vi "SpecAn ACP Configure.vi"(7 "Selector String":string, 8 "error in (no error)":errorcluster, 10 "ACP Common Configuration":T1={"Power Units"=0, "Averaging Enabled"=0, "Averaging Count"=10, "Averaging Type"=0, "FFT Window"=1, "FFT Padding"=1.0, "RBW Auto"=1, "RBW (Hz)"=10000.0, "RBW Filter Type"=1, "Sweep Time Auto"=1, "Sweep Time Interval (s)"=0.001, " Carrier Channel Configuration"=[], "Offset Channel Configuration"=[]} {"Offset Channel Configuration"."RRC Alpha" format="%.3g"; "Offset Channel Configuration"."RRC Enabled" items=["False", "True"]; "Offset Channel Configuration"."Relative Attenuation (dB)" format="%.2f"; "Offset Channel Configuration"."Offset Power Reference Carrier" items=["Closest", "Highest", "Composite", "Specific"]; "Offset Channel Configuration"."Offset Sideband" items=["Neg", "Pos", "Both"]; "Offset Channel Configuration"."Offset Frequency (Hz)" format="%.3p"; "Offset Channel Configuration"."Offset Enabled" items=["False", "True"]; "Offset Channel Configuration"."Integration Bandwidth (Hz)" format="%.3p"; "Carrier Channel Configuration"."RRC Alpha" format="%.3g"; "Carrier Channel Configuration"."RRC Enabled" items=["False", "True"]; "Carrier Channel Configuration"."Mode" items=["Passive", "Active"]; "Carrier Channel Configuration"."Frequency (Hz)" format="%.3p"; "Carrier Channel Configuration"."Integration Bandwidth (Hz)" format="%.3p"; "Sweep Time Interval (s)" format="%.2p"; "Sweep Time Auto" items=["False", "True"]; "RBW Filter Type" items=["FFT Based", "Gaussian", "Flat", "Synch Tuned - 4", "Synch Tuned - 5"]; "RBW (Hz)" format="%.3p"; "RBW Auto" items=["False", "True"]; "FFT Padding" format="%.2p"; "FFT Window" items=["None", "Flat Top", "Hanning", "Hamming", "Gaussian", "Blackman", "Blackman-Harris", "Kaiser-Bessel"]; "Averaging Type" items=["RMS", "Log", "Scalar", "Max", "Min", "Vector"]; "Averaging Enabled" items=["False", "True"]; "Power Units" items=["dBm", "dBm/Hz"]}, 11 "Instrument Handle In":refnum<k21>) -> (0 "error out":errorcluster, 3 "Instrument Handle Out":refnum<k21>)   [LabVIEW 2016, in "RFmxSpecAn.lvlib"]
uses:
  RFmxSpecAn.lvlib
  Typedefs/SpecAn ACP Common Configuration.ctl
  Typedefs/SpecAn ACP Carrier Channel Configuration.ctl
  Typedefs/SpecAn ACP Offset Channel Configuration.ctl
  <vilib>/RFmx/SpecAn/mx/RFmxSpecAn.llb/RFmxSpecAn Build Signal String.vi
  <vilib>/RFmx/RFInstr/mx/RFmxInstr.llb/RFmxInstr Build Signal String.vi
  <resource>/objmgr/RFmxSpecAn.rc
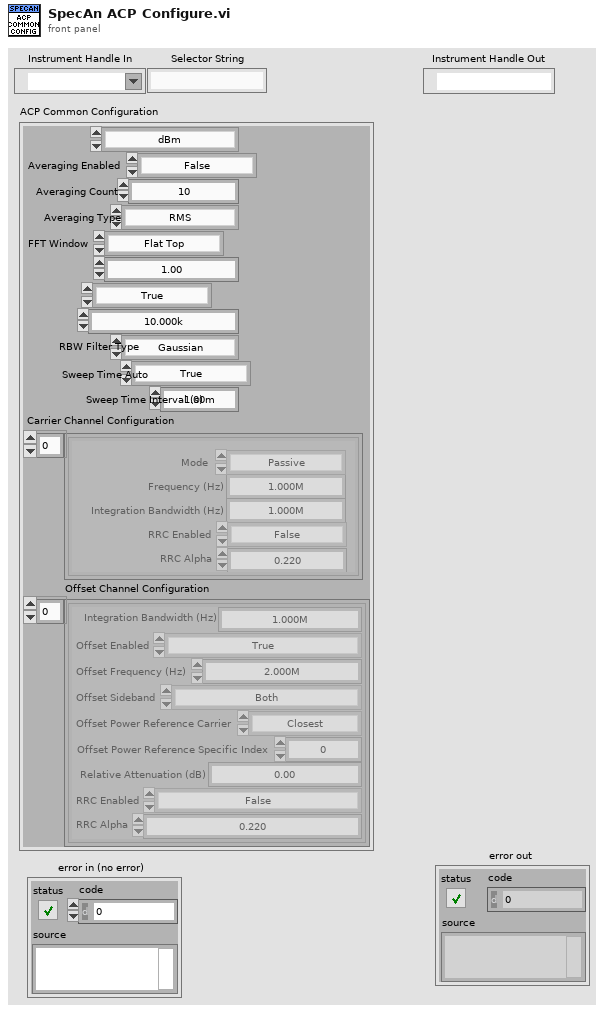
[diagram p1: front panel]
types:
  T1 = typedef "RFmxSpecAn.lvlib/SpecAn ACP Common Configuration.ctl" = cluster{"Power Units":i32, "Averaging Enabled":i32, "Averaging Count":i32, "Averaging Type":i32, "FFT Window":i32, "FFT Padding":dbl, "RBW Auto":i32, "RBW (Hz)":dbl, "RBW Filter Type":i32, "Sweep Time Auto":i32, "Sweep Time Interval (s)":dbl, " Carrier Channel Configuration":T2[], "Offset Channel Configuration":T3[]}
  T2 = typedef "RFmxSpecAn.lvlib/SpecAn ACP Carrier Channel Configuration.ctl" = cluster{"Frequency (Hz)":dbl, "Integration Bandwidth (Hz)":dbl, "Mode":i32, "RRC Enabled":i32, "RRC Alpha":dbl}
  T3 = typedef "RFmxSpecAn.lvlib/SpecAn ACP Offset Channel Configuration.ctl" = cluster{"Integration Bandwidth (Hz)":dbl, "Offset Enabled":i32, "Offset Frequency (Hz)":dbl, "Offset Sideband":i32, "Offset Power Reference Carrier":i32, "Offset Power Reference Specific Index":i32, "Relative Attenuation (dB)":dbl, "RRC Enabled":i32, "RRC Alpha":dbl}
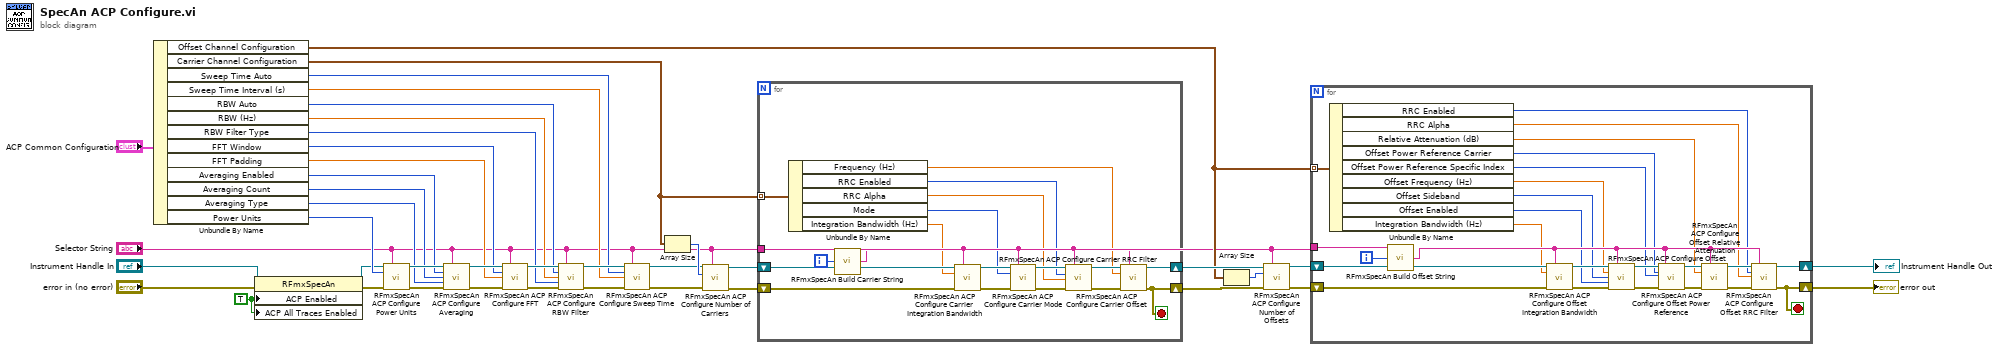
[diagram p0: block diagram]
diagram:
  w16 = TRUE ("ACP Enabled")
  n1 = Unbundle By Name("ACP Common Configuration") -> ("Offset Channel Configuration"=w4:T3[], "Carrier Channel Configuration"=w10:T2[], "Sweep Time Auto"=w22:i32, "Sweep Time Interval (s)"=w21:dbl, "RBW Auto"=w23:i32, "RBW (Hz)"=w24:dbl, "RBW Filter Type"=w25:i32, "FFT Window"=w27:i32, "FFT Padding"=w26:dbl, "Averaging Enabled"=w30:i32, "Averaging Count"=w29:i32, "Averaging Type"=w28:i32, "Power Units"=w31:i32)
  n2 = property class="RFmxSpecAn"(reference="Instrument Handle In", error in="error in (no error)", "ACP Enabled"=w16, "ACP All Traces Enabled"=w16) -> (reference out=w17:refnum<k21>, error out=w19:errorcluster)
  n3 = call <vilib>:"RFmxSpecAn ACP Configure Power Units.vi"("Instrument Handle In"=w17, "Selector String"="Selector String", "Power Units"=w31, "error in (no error)"=w19) -> ("Instrument Handle Out"=w36:refnum<k21>, "error out"=w35:errorcluster)  [unwired: 10 in]
  n4 = call <vilib>:"RFmxSpecAn ACP Configure Averaging.vi"("Instrument Handle In"=w36, "Selector String"="Selector String", "Averaging Enabled"=w30, "Averaging Count"=w29, "Averaging Type"=w28, "error in (no error)"=w35) -> ("Instrument Handle Out"=w34:refnum<k21>, "error out"=w40:errorcluster)  [unwired: 8 in]
  n5 = call <vilib>:"RFmxSpecAn ACP Configure FFT.vi"("Instrument Handle In"=w34, "Selector String"="Selector String", "FFT Window"=w27, "FFT Padding"=w26, "error in (no error)"=w40) -> ("Instrument Handle Out"=w38:refnum<k21>, "error out"=w37:errorcluster)  [unwired: 9 in]
  n6 = call <vilib>:"RFmxSpecAn ACP Configure RBW Filter.vi"("Instrument Handle In"=w38, "Selector String"="Selector String", "RBW Auto"=w23, "RBW (Hz)"=w24, "RBW Filter Type"=w25, "error in (no error)"=w37) -> ("Instrument Handle Out"=w33:refnum<k21>, "error out"=w39:errorcluster)  [unwired: 8 in]
  n7 = call <vilib>:"RFmxSpecAn ACP Configure Sweep Time.vi"("Instrument Handle In"=w33, "Selector String"="Selector String", "Sweep Time Auto"=w22, "Sweep Time Interval (s)"=w21, "error in (no error)"=w39) -> ("Instrument Handle Out"=w14:refnum<k21>, "error out"=w13:errorcluster)  [unwired: 9 in]
  n8 = Array Size(array=w10) -> (size(s)=w15:i32)
  n9 = call <vilib>:"RFmxSpecAn ACP Configure Number of Carriers.vi"("Instrument Handle In"=w14, "Selector String"="Selector String", "Number of Carriers"=w15, "error in (no error)"=w13) -> ("Instrument Handle Out"=w12:refnum<k21>, "error out"=w11:errorcluster)  [unwired: 10 in]
  n10 = for {
    tunnel: w10 -> [w51] mode=indexing
    shift-right: [w48] -> w5
    shift-left: w11 -> [w58]
    shift-right: [w50] -> w6
    shift-left: w12 -> [w59]
    tunnel: "Selector String" -> [w42]
    i -> [w49]
    stop <- w48 stop-if-true
    n11 = Unbundle By Name(w51) -> ("Frequency (Hz)"=w47:dbl, "RRC Enabled"=w46:i32, "RRC Alpha"=w45:dbl, "Mode"=w44:i32, "Integration Bandwidth (Hz)"=w43:dbl)
    n12 = call <vilib>:"RFmxSpecAn Build Carrier String.vi"("Signal Name"=w42, "Carrier Number"=w49) -> ("Carrier String"=w41:string)  [unwired: 13 in]
    n13 = call <vilib>:"RFmxSpecAn ACP Configure Carrier Integration Bandwidth.vi"("Instrument Handle In"=w59, "Selector String"=w41, "Integration Bandwidth (Hz)"=w43, "error in (no error)"=w58) -> ("Instrument Handle Out"=w57:refnum<k21>, "error out"=w56:errorcluster)  [unwired: 10 in]
    n14 = call <vilib>:"RFmxSpecAn ACP Configure Carrier Mode.vi"("Instrument Handle In"=w57, "Selector String"=w41, "Carrier Mode"=w44, "error in (no error)"=w56) -> ("Instrument Handle Out"=w55:refnum<k21>, "error out"=w54:errorcluster)  [unwired: 10 in]
    n15 = call <vilib>:"RFmxSpecAn ACP Configure Carrier RRC Filter.vi"("Instrument Handle In"=w55, "Selector String"=w41, "RRC Filter Enabled"=w46, "RRC Alpha"=w45, "error in (no error)"=w54) -> ("Instrument Handle Out"=w53:refnum<k21>, "error out"=w52:errorcluster)  [unwired: 9 in]
    n16 = call <vilib>:"RFmxSpecAn ACP Configure Carrier Offset.vi"("Instrument Handle In"=w53, "Selector String"=w41, "Carrier Frequency (Hz)"=w47, "error in (no error)"=w52) -> ("Instrument Handle Out"=w50:refnum<k21>, "error out"=w48:errorcluster)  [unwired: 10 in]
  }
  n17 = Array Size(array=w4) -> (size(s)=w7:i32)
  n18 = call <vilib>:"RFmxSpecAn ACP Configure Number of Offsets.vi"("Instrument Handle In"=w6, "Selector String"="Selector String", "Number of Offsets"=w7, "error in (no error)"=w5) -> ("Instrument Handle Out"=w9:refnum<k21>, "error out"=w8:errorcluster)  [unwired: 10 in]
  n19 = for {
    tunnel: w4 -> [w84] mode=indexing
    shift-right: [w70] -> w2
    shift-left: w8 -> [w82]
    shift-right: [w73] -> w3
    shift-left: w9 -> [w83]
    tunnel: "Selector String" -> [w60]
    i -> [w72]
    stop <- w70 stop-if-true
    n20 = Unbundle By Name(w84) -> ("RRC Enabled"=w69:i32, "RRC Alpha"=w68:dbl, "Relative Attenuation (dB)"=w67:dbl, "Offset Power Reference Carrier"=w66:i32, "Offset Power Reference Specific Index"=w65:i32, "Offset Frequency (Hz)"=w64:dbl, "Offset Sideband"=w63:i32, "Offset Enabled"=w62:i32, "Integration Bandwidth (Hz)"=w61:dbl)
    n21 = call <vilib>:"RFmxSpecAn Build Offset String.vi"("Signal Name"=w60, "Offset Number"=w72) -> ("Offset String"=w71:string)  [unwired: 13 in]
    n22 = call <vilib>:"RFmxSpecAn ACP Configure Offset Integration Bandwidth.vi"("Instrument Handle In"=w83, "Selector String"=w71, "Integration Bandwidth (Hz)"=w61, "error in (no error)"=w82) -> ("Instrument Handle Out"=w81:refnum<k21>, "error out"=w80:errorcluster)  [unwired: 10 in]
    n23 = call <vilib>:"RFmxSpecAn ACP Configure Offset.vi"("Instrument Handle In"=w81, "Selector String"=w71, "Offset Frequency (Hz)"=w64, "Offset Sideband"=w63, "Offset Enabled"=w62, "error in (no error)"=w80) -> ("Instrument Handle Out"=w79:refnum<k21>, "error out"=w78:errorcluster)  [unwired: 8 in]
    n24 = call <vilib>:"RFmxSpecAn ACP Configure Offset Power Reference.vi"("Instrument Handle In"=w79, "Selector String"=w71, "Offset Power Reference Carrier"=w66, "Offset Power Reference Specific"=w65, "error in (no error)"=w78) -> ("Instrument Handle Out"=w77:refnum<k21>, "error out"=w76:errorcluster)  [unwired: 9 in]
    n25 = call <vilib>:"RFmxSpecAn ACP Configure Offset Relative Attenuation.vi"("Instrument Handle In"=w77, "Selector String"=w71, "Relative Attenuation (dB)"=w67, "error in (no error)"=w76) -> ("Instrument Handle Out"=w75:refnum<k21>, "error out"=w74:errorcluster)  [unwired: 10 in]
    n26 = call <vilib>:"RFmxSpecAn ACP Configure Offset RRC Filter.vi"("Instrument Handle In"=w75, "Selector String"=w71, "RRC Filter Enabled"=w69, "RRC Alpha"=w68, "error in (no error)"=w74) -> ("Instrument Handle Out"=w73:refnum<k21>, "error out"=w70:errorcluster)  [unwired: 9 in]
  }
  "Instrument Handle Out" <- w3
  "error out" <- w2
